vi "test-Mecanum-Kinematics-Test2.vi"() -> (3 "All tests passed":bool)   [LabVIEW 2019]
uses:
  <vilib>/Rock Robotics/WPI/ThirdParty/JAS_Junk/TrajLib/Trajectory_Library.lvlib
panel:
  out "Test 12":bool
  out "Test 10":bool
  out "Test 8":bool
  out "Test 6":bool
  out "Test 4":bool
  out "Test 2":bool
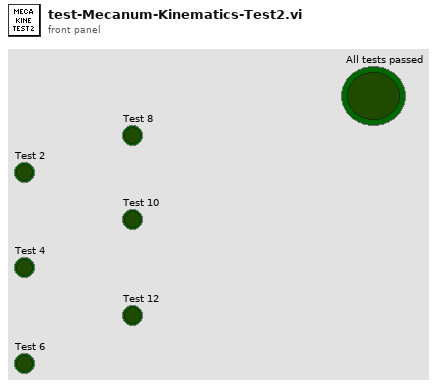
[diagram p1: front panel]
types:
  T1 = typedef "Trajectory_Library.lvlib/TRANSLATION2D.ctl" = cluster{"X":dbl, "Y":dbl}
  T2 = typedef "Trajectory_Library.lvlib/MECA_WHEEL_POSITIONS.ctl" = cluster{"FrontLeft":dbl, "FrontRight":dbl, "RearLeft":dbl, "RearRight":dbl, "P":bool}
  T3 = typedef "Trajectory_Library.lvlib/MECA_DRIVE_KINEMATICS.ctl" = cluster{"FrontLeft":T1, "FrontRight":T1, "RearLeft":T1, "RearRight":T1, "InverseKinematics":T4, "ForwardKinematics":T4, "PrevCoR":T1}
  T4 = typedef "NI_Matrix.lvlib/RealMatrix.ctl" = dbl[][]
  T5 = typedef "Trajectory_Library.lvlib/TWIST2D.ctl" = cluster{"dX":dbl, "dY":dbl, "dTHETA":dbl}
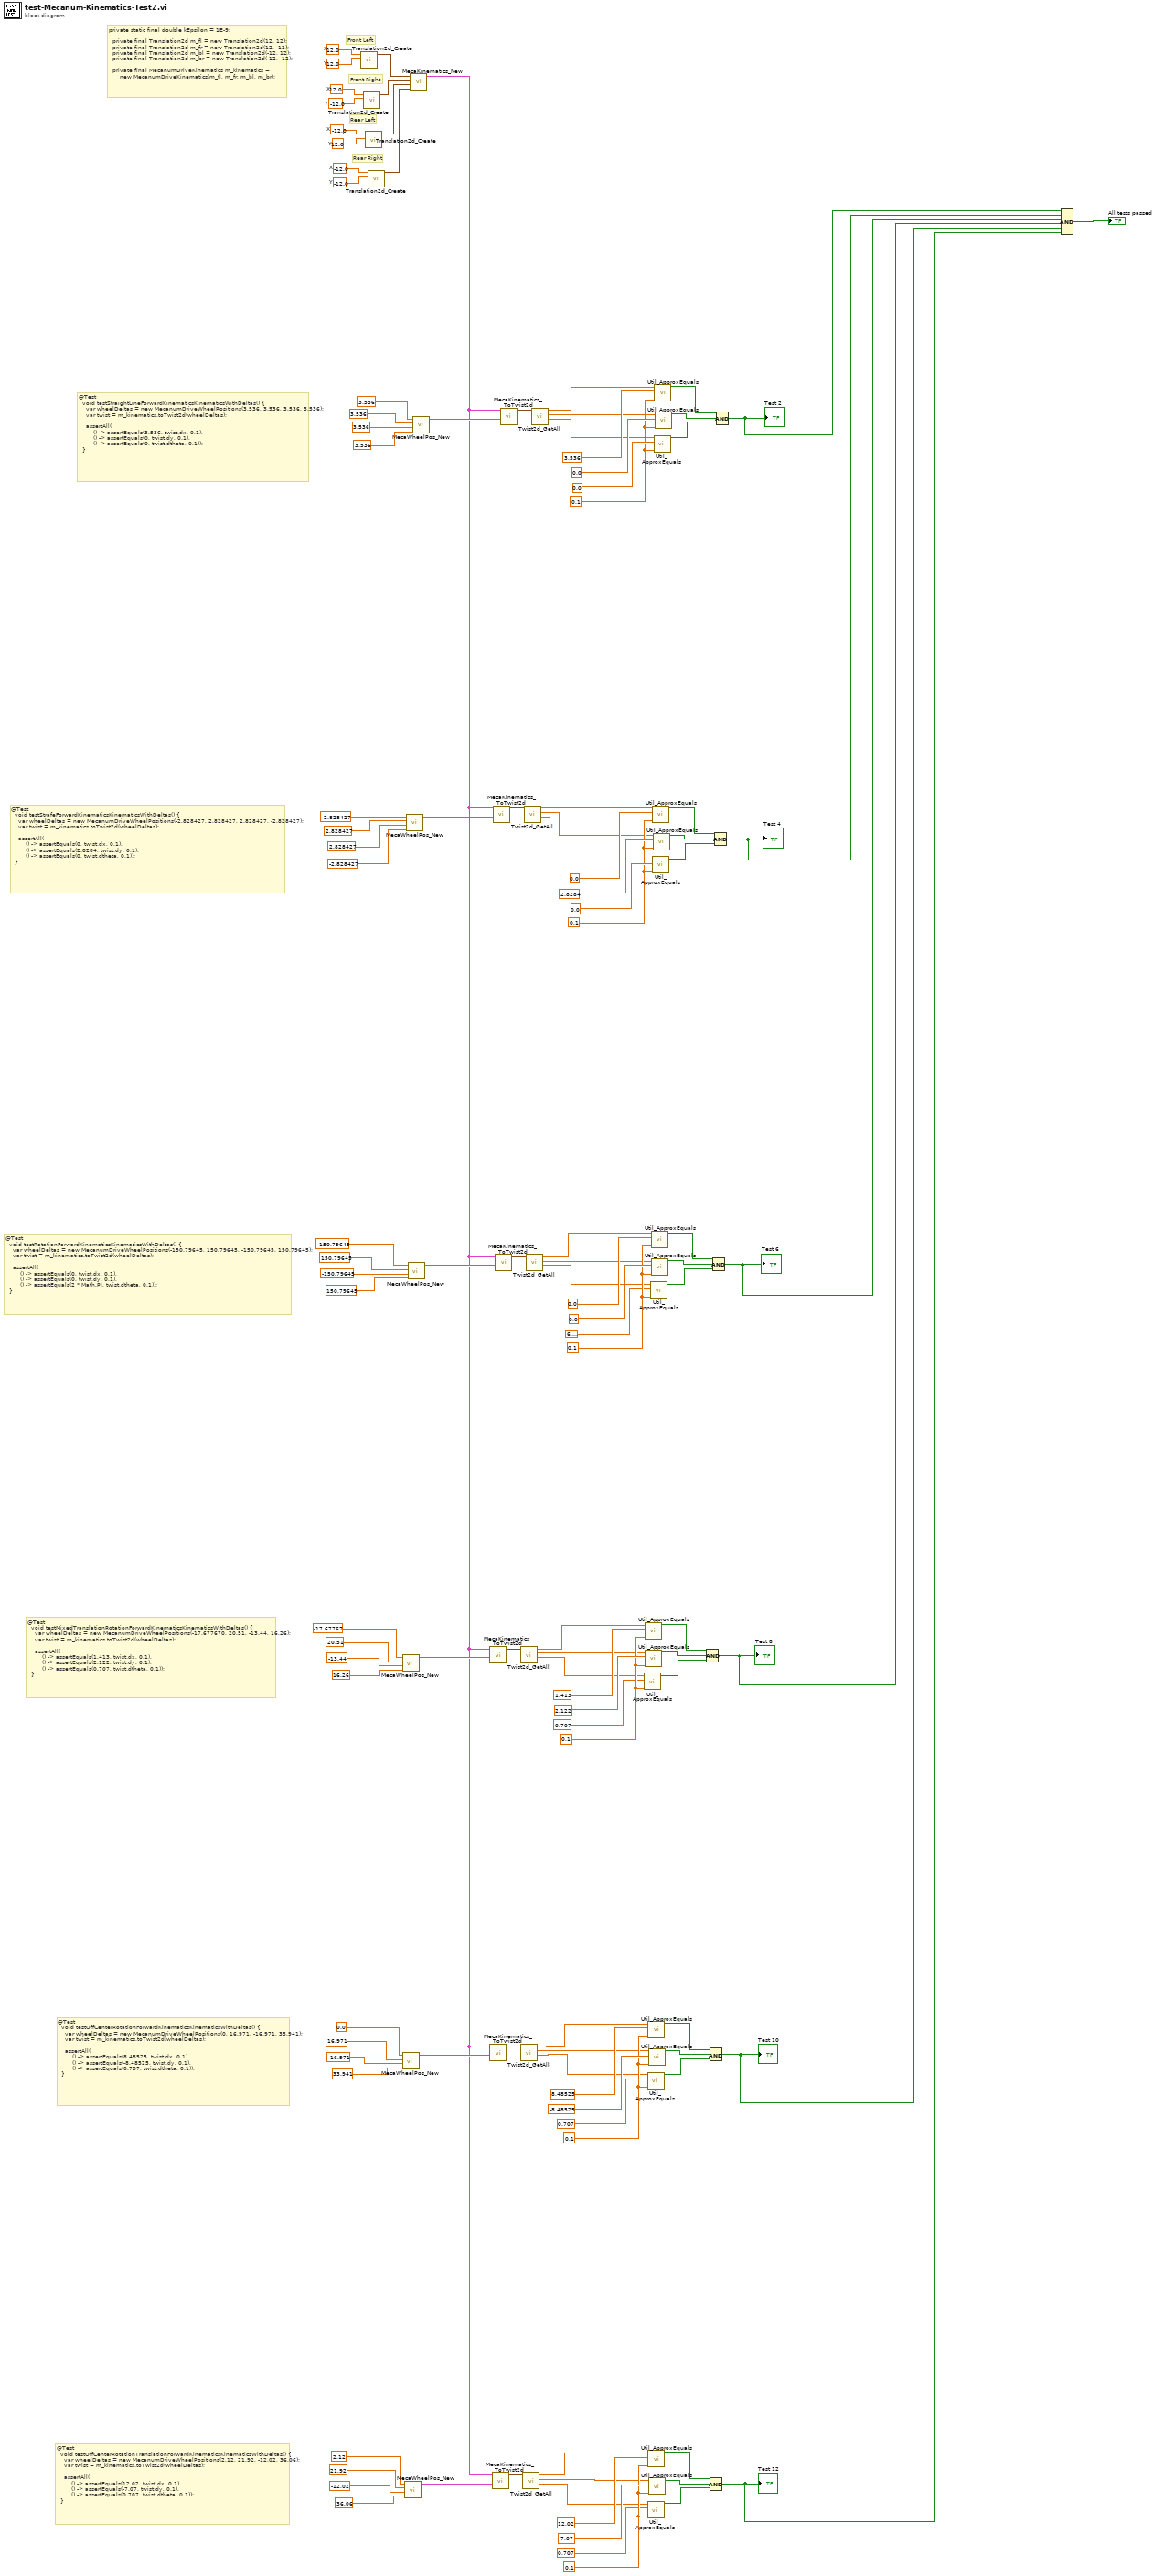
[diagram p0: block diagram]
diagram:
  w58 = 0.1 ("Tolerance")
  w66 = 0.1 ("Tolerance")
  w76 = 0.1 ("Tolerance")
  w83 = 0.1 ("Tolerance")
  w89 = 0.1 ("Tolerance")
  w96 = 0.1 ("Tolerance")
  w111 = -12.0  # X
  w110 = -12.0  # Y
  w109 = -12.0  # X
  w108 = 12.0  # Y
  w107 = 12.0  # X
  w106 = -12.0  # Y
  w105 = 12.0  # X
  w104 = 12.0  # Y
  # "@Test\n  void testOffCenterRotationTranslationForwardKinematicsKinematicsWithDeltas() {\n    var wheelDeltas = new MecanumDriveWheelPositions(2.12, 21.92, -12.02, 36.06);\n    var twist = m_kinematics.toTwist2d(wheelDeltas);\n\n    assertAll(\n        () -> assertEquals(12.02, twist.dx, 0.1),\n        () -> assertEquals(-7.07, twist.dy, 0.1),\n        () -> assertEquals(0.707, twist.dtheta, 0.1));\n  }"
  # "@Test\n  void testOffCenterRotationForwardKinematicsKinematicsWithDeltas() {\n    var wheelDeltas = new MecanumDriveWheelPositions(0, 16.971, -16.971, 33.941);\n    var twist = m_kinematics.toTwist2d(wheelDeltas);\n\n    assertAll(\n        () -> assertEquals(8.48525, twist.dx, 0.1),\n        () -> assertEquals(-8.48525, twist.dy, 0.1),\n        () -> assertEquals(0.707, twist.dtheta, 0.1));\n  }"
  # "@Test\n  void testMixedTranslationRotationForwardKinematicsKinematicsWithDeltas() {\n    var wheelDeltas = new MecanumDriveWheelPositions(-17.677670, 20.51, -13.44, 16.26);\n    var twist = m_kinematics.toTwist2d(wheelDeltas);\n\n    assertAll(\n        () -> assertEquals(1.413, twist.dx, 0.1),\n        () -> assertEquals(2.122, twist.dy, 0.1),\n        () -> assertEquals(0.707, twist.dtheta, 0.1));\n  }"
  # "@Test\n  void testRotationForwardKinematicsKinematicsWithDeltas() {\n    var wheelDeltas = new MecanumDriveWheelPositions(-150.79645, 150.79645, -150.79645, 150.79645);\n    var twist = m_kinematics.toTwist2d(wheelDeltas);\n\n    assertAll(\n        () -> assertEquals(0, twist.dx, 0.1),\n        () -> assertEquals(0, twist.dy, 0.1),\n        () -> assertEquals(2 * Math.PI, twist.dtheta, 0.1));\n  }"
  # "@Test\n  void testStrafeForwardKinematicsKinematicsWithDeltas() {\n    var wheelDeltas = new MecanumDriveWheelPositions(-2.828427, 2.828427, 2.828427, -2.828427);\n    var twist = m_kinematics.toTwist2d(wheelDeltas);\n\n    assertAll(\n        () -> assertEquals(0, twist.dx, 0.1),\n        () -> assertEquals(2.8284, twist.dy, 0.1),\n        () -> assertEquals(0, twist.dtheta, 0.1));\n  }"
  # "@Test\n  void testStraightLineForwardKinematicsKinematicsWithDeltas() {\n    var wheelDeltas = new MecanumDriveWheelPositions(3.536, 3.536, 3.536, 3.536);\n    var twist = m_kinematics.toTwist2d(wheelDeltas);\n\n    assertAll(\n        () -> assertEquals(3.536, twist.dx, 0.1),\n        () -> assertEquals(0, twist.dy, 0.1),\n        () -> assertEquals(0, twist.dtheta, 0.1));\n  }"
  # "Rear Right"
  # "Rear Left"
  # "Front Right"
  # "Front Left"
  # "private static final double kEpsilon = 1E-9;\n\n  private final Translation2d m_fl = new Translation2d(12, 12);\n  private final Translation2d m_fr = new Translation2d(12, -12);\n  private final Translation2d m_bl = new Translation2d(-12, 12);\n  private final Translation2d m_br = new Translation2d(-12, -12);\n\n  private final MecanumDriveKinematics m_kinematics =\n      new MecanumDriveKinematics(m_fl, m_fr, m_bl, m_br);"
  n1 = call <vilib>:"Translation2d_Create.vi"("Y"=w104, "X"=w105) -> ("TRANSLATION"=w112:T1)  [unwired: 9 in]
  n2 = call <vilib>:"Translation2d_Create.vi"("Y"=w106, "X"=w107) -> ("TRANSLATION"=w113:T1)  [unwired: 9 in]
  n3 = call <vilib>:"Translation2d_Create.vi"("Y"=w108, "X"=w109) -> ("TRANSLATION"=w114:T1)  [unwired: 9 in]
  n4 = call <vilib>:"Translation2d_Create.vi"("Y"=w110, "X"=w111) -> ("TRANSLATION"=w115:T1)  [unwired: 9 in]
  n5 = call <vilib>:"MecaWheelPos_New.vi"("RearRightPosition"=16.26 ("RearRightSpeed"), "RearLeftPosition"=-13.44 ("RearLeftSpeed"), "FrontRightPosition"=20.51 ("FrontRightSpeed"), "FrontLeftPosition"=-17.67767 ("FrontLeftSpeed")) -> ("MECA_WHEEL_POSITIONS"=w31:T2)  [unwired: 7 in]
  n6 = call <vilib>:"MecaWheelPos_New.vi"("RearRightPosition"=33.941 ("RearRightSpeed"), "RearLeftPosition"=-16.971 ("RearLeftSpeed"), "FrontRightPosition"=16.971 ("FrontRightSpeed"), "FrontLeftPosition"=0.0 ("FrontLeftSpeed")) -> ("MECA_WHEEL_POSITIONS"=w23:T2)  [unwired: 7 in]
  n7 = call <vilib>:"MecaWheelPos_New.vi"("RearRightPosition"=36.06 ("RearRightSpeed"), "RearLeftPosition"=-12.02 ("RearLeftSpeed"), "FrontRightPosition"=21.92 ("FrontRightSpeed"), "FrontLeftPosition"=2.12 ("FrontLeftSpeed")) -> ("MECA_WHEEL_POSITIONS"=w15:T2)  [unwired: 7 in]
  n8 = call <vilib>:"MecaWheelPos_New.vi"("RearRightPosition"=-2.828427 ("RearRightSpeed"), "RearLeftPosition"=2.828427 ("RearLeftSpeed"), "FrontRightPosition"=2.828427 ("FrontRightSpeed"), "FrontLeftPosition"=-2.828427 ("FrontLeftSpeed")) -> ("MECA_WHEEL_POSITIONS"=w47:T2)  [unwired: 7 in]
  n9 = call <vilib>:"MecaWheelPos_New.vi"("RearRightPosition"=150.79645 ("RearRightSpeed"), "RearLeftPosition"=-150.79645 ("RearLeftSpeed"), "FrontRightPosition"=150.79645 ("FrontRightSpeed"), "FrontLeftPosition"=-150.79645 ("FrontLeftSpeed")) -> ("MECA_WHEEL_POSITIONS"=w39:T2)  [unwired: 7 in]
  n10 = call <vilib>:"MecaKinematics_New.vi"("RearRight"=w115, "RearLeft"=w114, "FrontRight"=w113, "FrontLeft"=w112) -> ("MECA_DRIVE_KINEMATICS"=w14:T3)  [unwired: 7 in]
  n11 = call <vilib>:"MecaWheelPos_New.vi"("RearRightPosition"=3.536, "RearLeftPosition"=3.536, "FrontRightPosition"=3.536, "FrontLeftPosition"=3.536) -> ("MECA_WHEEL_POSITIONS"=w51:T2)  [unwired: 7 in]
  n12 = call <vilib>:"MecaKinematics_ToTwist2d.vi"("Wheel Deltat Positions"=w31, "in MECA_DRIVE_KINEMATICS"=w14) -> ("Twist2d"=w4:T5)  [unwired: 9 in]
  n13 = call <vilib>:"MecaKinematics_ToTwist2d.vi"("Wheel Deltat Positions"=w23, "in MECA_DRIVE_KINEMATICS"=w14) -> ("Twist2d"=w2:T5)  [unwired: 9 in]
  n14 = call <vilib>:"MecaKinematics_ToTwist2d.vi"("Wheel Deltat Positions"=w15, "in MECA_DRIVE_KINEMATICS"=w14) -> ("Twist2d"=w1:T5)  [unwired: 9 in]
  n15 = call <vilib>:"MecaKinematics_ToTwist2d.vi"("Wheel Deltat Positions"=w47, "in MECA_DRIVE_KINEMATICS"=w14) -> ("Twist2d"=w5:T5)  [unwired: 9 in]
  n16 = call <vilib>:"MecaKinematics_ToTwist2d.vi"("Wheel Deltat Positions"=w39, "in MECA_DRIVE_KINEMATICS"=w14) -> ("Twist2d"=w3:T5)  [unwired: 9 in]
  n17 = call <vilib>:"MecaKinematics_ToTwist2d.vi"("Wheel Deltat Positions"=w51, "in MECA_DRIVE_KINEMATICS"=w14) -> ("Twist2d"=w6:T5)  [unwired: 9 in]
  n18 = call <vilib>:"Twist2d_GetAll.vi"("TWIST"=w4) -> ("dTHETA"=w29:dbl, "dY"=w28:dbl, "dX"=w30:dbl)  [unwired: 8 in]
  n19 = call <vilib>:"Twist2d_GetAll.vi"("TWIST"=w2) -> ("dTHETA"=w20:dbl, "dY"=w21:dbl, "dX"=w22:dbl)  [unwired: 8 in]
  n20 = call <vilib>:"Twist2d_GetAll.vi"("TWIST"=w1) -> ("dTHETA"=w11:dbl, "dY"=w12:dbl, "dX"=w13:dbl)  [unwired: 8 in]
  n21 = call <vilib>:"Twist2d_GetAll.vi"("TWIST"=w5) -> ("dTHETA"=w40:dbl, "dY"=w41:dbl, "dX"=w42:dbl)  [unwired: 8 in]
  n22 = call <vilib>:"Twist2d_GetAll.vi"("TWIST"=w3) -> ("dTHETA"=w32:dbl, "dY"=w33:dbl, "dX"=w34:dbl)  [unwired: 8 in]
  n23 = call <vilib>:"Twist2d_GetAll.vi"("TWIST"=w6) -> ("dTHETA"=w48:dbl, "dY"=w49:dbl, "dX"=w50:dbl)  [unwired: 8 in]
  n24 = call <vilib>:"Util_ApproxEquals.vi"("Tolerance"=w76, "Value 2"=0.707, "Value 1"=w29) -> ("ApproxEquals"=w77:bool)  [unwired: 8 in]
  n25 = call <vilib>:"Util_ApproxEquals.vi"("Tolerance"=w76, "Value 2"=1.413, "Value 1"=w30) -> ("ApproxEquals"=w79:bool)  [unwired: 8 in]
  n26 = call <vilib>:"Util_ApproxEquals.vi"("Tolerance"=w76, "Value 2"=2.122, "Value 1"=w28) -> ("ApproxEquals"=w78:bool)  [unwired: 8 in]
  n27 = call <vilib>:"Util_ApproxEquals.vi"("Tolerance"=w66, "Value 2"=0.707, "Value 1"=w20) -> ("ApproxEquals"=w67:bool)  [unwired: 8 in]
  n28 = call <vilib>:"Util_ApproxEquals.vi"("Tolerance"=w58, "Value 2"=0.707, "Value 1"=w11) -> ("ApproxEquals"=w59:bool)  [unwired: 8 in]
  n29 = call <vilib>:"Util_ApproxEquals.vi"("Tolerance"=w66, "Value 2"=8.48525, "Value 1"=w22) -> ("ApproxEquals"=w69:bool)  [unwired: 8 in]
  n30 = call <vilib>:"Util_ApproxEquals.vi"("Tolerance"=w58, "Value 2"=12.02, "Value 1"=w13) -> ("ApproxEquals"=w61:bool)  [unwired: 8 in]
  n31 = call <vilib>:"Util_ApproxEquals.vi"("Tolerance"=w66, "Value 2"=-8.48525, "Value 1"=w21) -> ("ApproxEquals"=w68:bool)  [unwired: 8 in]
  n32 = call <vilib>:"Util_ApproxEquals.vi"("Tolerance"=w58, "Value 2"=-7.07, "Value 1"=w12) -> ("ApproxEquals"=w60:bool)  [unwired: 8 in]
  n33 = call <vilib>:"Util_ApproxEquals.vi"("Tolerance"=w83, "Value 2"=6.283185307179586, "Value 1"=w32) -> ("ApproxEquals"=w84:bool)  [unwired: 8 in]
  n34 = call <vilib>:"Util_ApproxEquals.vi"("Tolerance"=w83, "Value 2"=0.0, "Value 1"=w34) -> ("ApproxEquals"=w86:bool)  [unwired: 8 in]
  n35 = call <vilib>:"Util_ApproxEquals.vi"("Tolerance"=w83, "Value 2"=0.0, "Value 1"=w33) -> ("ApproxEquals"=w85:bool)  [unwired: 8 in]
  n36 = call <vilib>:"Util_ApproxEquals.vi"("Tolerance"=w89, "Value 2"=0.0, "Value 1"=w40) -> ("ApproxEquals"=w90:bool)  [unwired: 8 in]
  n37 = call <vilib>:"Util_ApproxEquals.vi"("Tolerance"=w89, "Value 2"=0.0, "Value 1"=w42) -> ("ApproxEquals"=w92:bool)  [unwired: 8 in]
  n38 = call <vilib>:"Util_ApproxEquals.vi"("Tolerance"=w89, "Value 2"=2.8284, "Value 1"=w41) -> ("ApproxEquals"=w91:bool)  [unwired: 8 in]
  n39 = call <vilib>:"Util_ApproxEquals.vi"("Tolerance"=w96, "Value 2"=0.0, "Value 1"=w48) -> ("ApproxEquals"=w98:bool)  [unwired: 8 in]
  n40 = call <vilib>:"Util_ApproxEquals.vi"("Tolerance"=w96, "Value 2"=3.536, "Value 1"=w50) -> ("ApproxEquals"=w100:bool)  [unwired: 8 in]
  n41 = call <vilib>:"Util_ApproxEquals.vi"("Tolerance"=w96, "Value 2"=0.0, "Value 1"=w49) -> ("ApproxEquals"=w99:bool)  [unwired: 8 in]
  n42 = Compound Arithmetic op=AND(w79, w78, w77) -> (w72:bool)
  "Test 8" <- w72
  n43 = Compound Arithmetic op=AND(w69, w68, w67) -> (w64:bool)
  "Test 10" <- w64
  n44 = Compound Arithmetic op=AND(w61, w60, w59) -> (w56:bool)
  "Test 12" <- w56
  n45 = Compound Arithmetic op=AND(w86, w85, w84) -> (w73:bool)
  "Test 6" <- w73
  n46 = Compound Arithmetic op=AND(w92, w91, w90) -> (w74:bool)
  "Test 4" <- w74
  n47 = Compound Arithmetic op=AND(w100, w99, w98) -> (w97:bool)
  "Test 2" <- w97
  n48 = Compound Arithmetic op=AND(w97, w74, w73, w72, w64, w56) -> (→"All tests passed":bool)
